vi "LVIS_LaunchLog.vi"(8 "Error In":errorcluster) -> (0 "Error Out":errorcluster)   [LabVIEW 2015]
doc: "If enabled in the LVIS_Settings file, launches the Event Log panel."
uses:
  Globals/LVIS_DcGlobals.vi
  Globals/LVIS_IsGlobal.vi
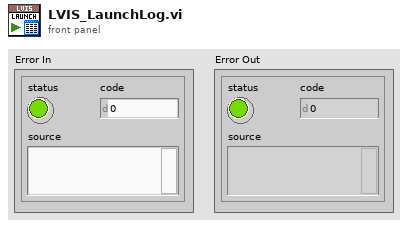
[diagram p1: front panel]
types:
  T1 = enum32{"Invalid", "Standard", "Closed", "Hidden", "Minimized", "Maximized"}
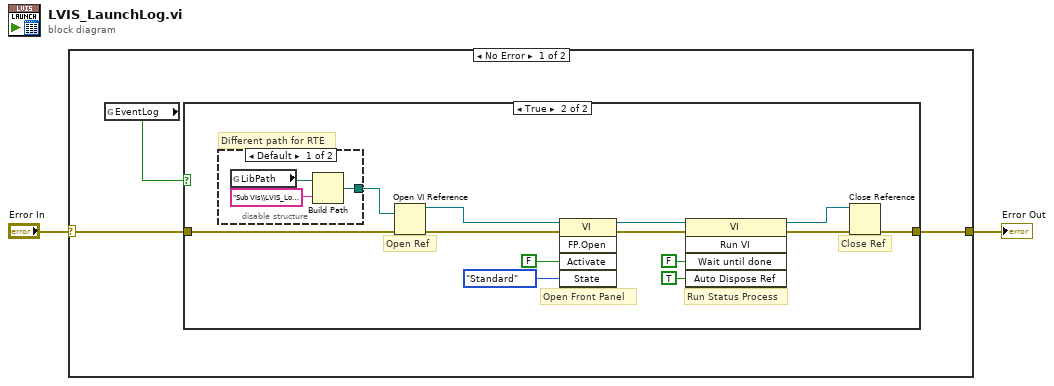
[diagram p0: block diagram]
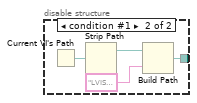
[diagram p3: hidden frame]
diagram:
  n1 = case shown="No Error" "Error In" {
    selector: "Error In" -> [w5 w27]
    tunnel: [w4 w27] -> w1
    frame No Error {
      n2 = global read "LVIS_DcGlobals.vi" "EventLog"() -> (w3:bool)
      n3 = case shown="True" w3 {
        tunnel: w5 -> [w6 w19]
        tunnel: [w6 w18] -> w4
        frame False {
          # "The event log is not enabled"
        }
        frame True {
          # "Different path for RTE"
          # "Run Status Process"
          # "Open Front Panel"
          # "Close Ref"
          # "Open Ref"
          n4 = disable-structure shown="Default" {
            disable-tunnel: [w21 w23] -> w7
            frame condition #0 (active) {
              n5 = global read "LVIS_IsGlobal.vi" "LibPath"() -> (w22:path)
              n6 = Build Path(base path=w22, name or relative path="Sub VIs\\LVIS_Log.vi") -> (appended path=w21:path)
            }
            frame condition #1 {
              n7 = Current VI's Path() -> (path=w26:path)
              n8 = Strip Path(path=w26) -> (stripped path=w25:path)  [unwired: 1 out]
              n9 = Build Path(base path=w25, name or relative path="LVIS_Log.vi") -> (appended path=w23:path)
            }
          }
          n10 = Open VI Reference(vi path=w7, error in (no error)=w19) -> (vi reference=w8:refnum<vi>, error out=w9:errorcluster)  [unwired: 4 in]
          n11 = invoke class="VI" method="FP.Open"(reference=w8, error in=w9, "Activate"=FALSE ("Activate?"), "State"=T1."Standard") -> (reference out=w12:refnum<vi>, error out=w13:errorcluster)  [unwired: 1 in, 3 out]
          n12 = invoke class="VI" method="Run VI"(reference=w12, error in=w13, "Wait until done"=FALSE ("Wait Until Done"), "Auto Dispose Ref"=TRUE ("Auto Dispose Reference")) -> (reference out=w16:refnum<vi>, error out=w17:errorcluster)  [unwired: 1 in, 3 out]
          n13 = Close Reference(reference=w16, error in (no error)=w17) -> (error out=w18:errorcluster)
        }
      }
    }
    frame Error {
    }
  }
  "Error Out" <- w1
